vi "Triangular Matrix to array.vi"(8 "index second subarray":i32, 9 "index first subarray":i32, 11 "Array":dbl[][](array[numeric])) -> (0 "Array second":dbl[](array[numeric]), 3 "Array first":dbl[](array[numeric]))   [LabVIEW 2014]
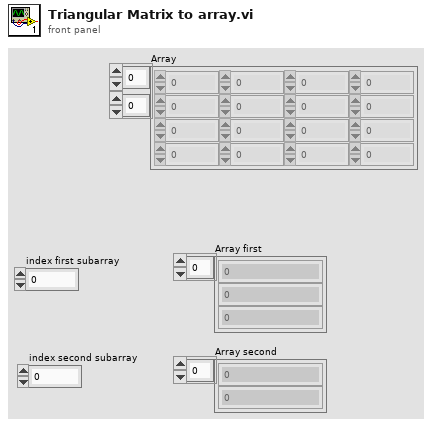
[diagram p1: front panel]
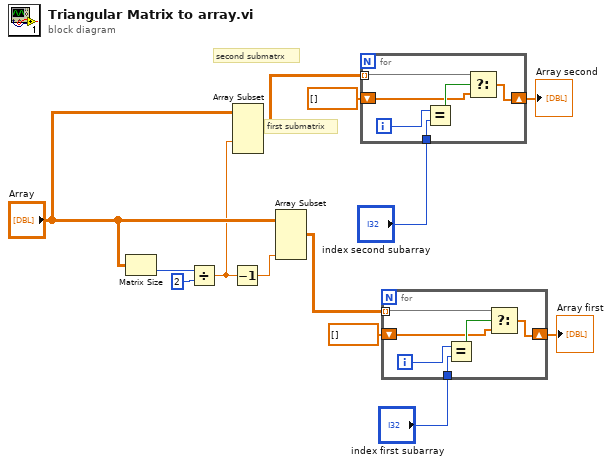
[diagram p0: block diagram]
diagram:
  # "second submatrx"
  # "first submatrix"
  n1 = Matrix Size(0:"Array") -> (2:w13:i32)  [unwired: 1 out]
  n2 = Divide(x=w13, y=2) -> (x/y=w10:dbl)
  n3 = Decrement(x=w10) -> (x-1=w9:dbl)
  n4 = Array Subset(array="Array", index (col)=w10) -> (w8:dbl[][])  [unwired: 3 in]
  n5 = Array Subset(array="Array", length (col)=w9) -> (w1:dbl[][])  [unwired: 3 in]
  n6 = for {
    tunnel: w8 -> [w18] mode=indexing
    shift-right: [w16] -> w6
    shift-left: dbl[] [] -> [w14]
    tunnel: "index second subarray" -> [w15]
    i -> [w19]
    n7 = Equal?(x=w19, y=w15) -> (x = y?=w17:bool)
    n8 = Select(t=w18, s=w17, f=w14) -> (s? t:f=w16:dbl[])
  }
  "Array second" <- w6
  n9 = for {
    tunnel: w1 -> [w24] mode=indexing
    shift-right: [w22] -> w3
    shift-left: dbl[] [] -> [w20]
    tunnel: "index first subarray" -> [w21]
    i -> [w25]
    n10 = Equal?(x=w25, y=w21) -> (x = y?=w23:bool)
    n11 = Select(t=w24, s=w23, f=w20) -> (s? t:f=w22:dbl[])
  }
  "Array first" <- w3
